vi "GetCircleResultValue.vi"(8 "error in (no error)":errorcluster, 9 "data":T2 {"ROI Descriptor out"."Contours"."Type" items=["No Selection", "Point", "Line", "Rectangle", "Oval", "Polygon", "Freehand Region", "Annulus", "Unused2", "Unused3", "Broken Line", "Freehand Line", "Rotated Rectangle"]; "ROI Descriptor out"."Contours"."Type" items=["No Selection", "Point", "Line", "Rectangle", "Oval", "Polygon", "Freehand Region", "Annulus", "Unused2", "Unused3", "Broken Line", "Freehand Line", "Rotated Rectangle"]}, 11 "Analysis_Circle_Parameter":T3={"ROI Descriptor"={"Global Rectangle"=[], "Contours"=[]}, "Options"={"Search  Direction"=0, "Edge Options"={"Edge Polarity"=0, "Kernel Size"=3, "Width"=3, "Minimum Edge Strength"=10.0, "Interpolation Type"=enum."Bilinear Fixed", "Data Processing Method"=enum."Average"}, "Show Search Area"=FALSE, "Show Search Lines"=FALSE, "Show Edges Found"=FALSE, "Show Result"=TRUE, "Search Area Color"=65280, "Search Lines Color"=255, "Edge Locations Color"=16776960, "Result Color"=16711680, "Overlay Group Name"=""}, "Circle Fit Options"={"Process"=enum."Get First Edge", "Step Size"=3.0, "Max Pixel Radius"=3}} {"Options"."Search  Direction" items=["Outside to Inside", "Inside to Outside"]; "Options"."Edge Options"."Edge Polarity" items=["All Edges", "Rising Edges", "Falling Edges"]; "Options"."Edge Options"."Minimum Edge Strength" format="%.2f"; "Options"."Edge Options"."Width" step=2; "Options"."Edge Options"."Kernel Size" step=2}) -> (0 "error out":errorcluster, 3 "ResultValues":string[](array[string]))   [LabVIEW 2019]
uses:
  Controls/Circle/Analysis_Circle_Parameter.ctl
  <vilib>/vision/Measure.llb/Edge Options.ctl
  <vilib>/vision/Measure.llb/Edge Polarity.ctl
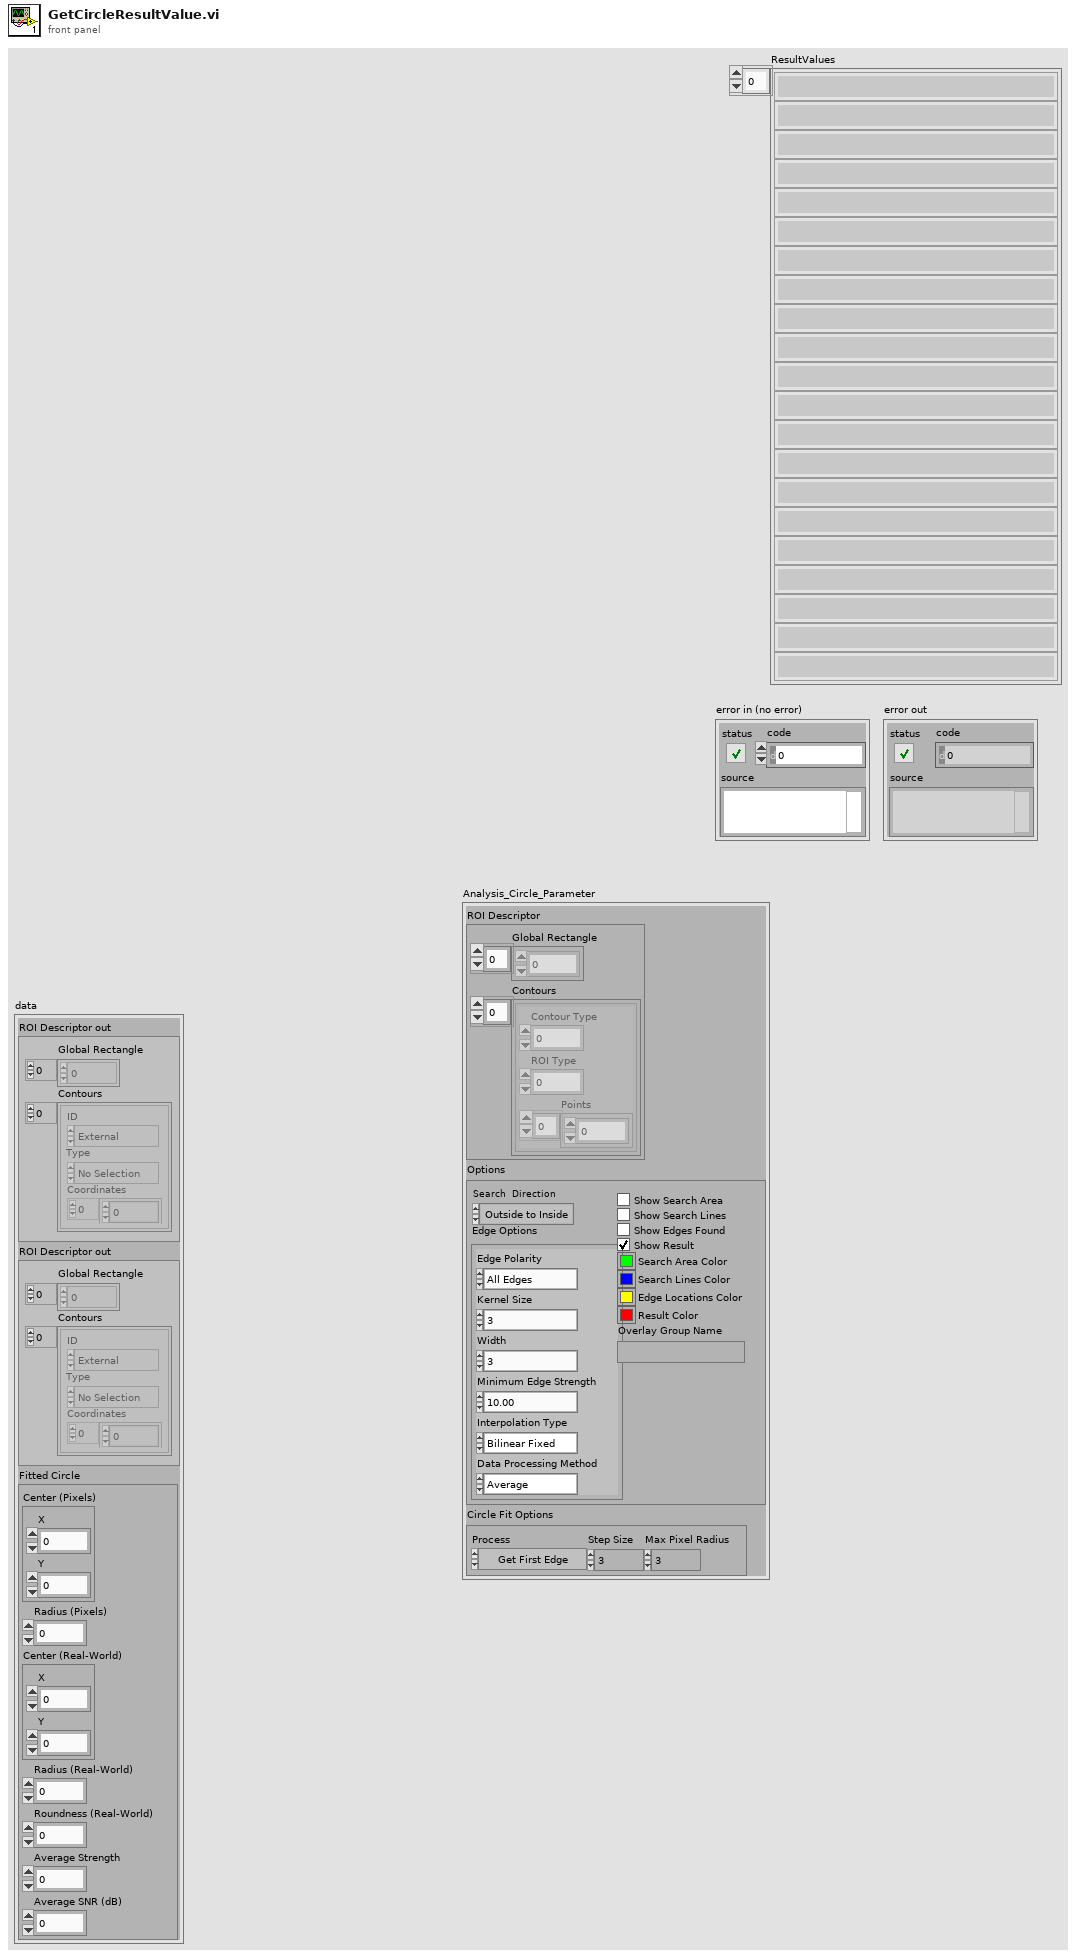
[diagram p1: front panel]
types:
  T1 = typedef "ROI Descriptor" = cluster{"Global Rectangle":i32[], "Contours":cluster{"ID":enum32{"External", "Internal"}, "Type":u32, "Coordinates":i32[]}[]}
  T2 = cluster{"ROI Descriptor out":T1, "ROI Descriptor out":T1, "Fitted Circle":cluster{"Center (Pixels)":cluster{"X":sgl, "Y":sgl}, "Radius (Pixels)":dbl, "Center (Real-World)":cluster{"X":sgl, "Y":sgl}, "Radius (Real-World)":dbl, "Roundness (Real-World)":dbl, "Average Strength":dbl, "Average SNR (dB)":dbl}}
  T3 = typedef "Analysis_Circle_Parameter.ctl" = cluster{"ROI Descriptor":cluster{"Global Rectangle":i32[], "Contours":cluster{"Contour Type":u32, "ROI Type":u32, "Points":i32[]}[]}, "Options":cluster{"Search  Direction":u32, "Edge Options":T4, "Show Search Area":bool, "Show Search Lines":bool, "Show Edges Found":bool, "Show Result":bool, "Search Area Color":u32, "Search Lines Color":u32, "Edge Locations Color":u32, "Result Color":u32, "Overlay Group Name":string}, "Circle Fit Options":cluster{"Process":enum16{"Get First Edge", "Get First + Last Edge", "Get All Edges", "Get Best Edge"}, "Step Size":dbl, "Max Pixel Radius":i32}}
  T4 = typedef "Edge Options.ctl" = cluster{"Edge Polarity":T5, "Kernel Size":u32, "Width":u32, "Minimum Edge Strength":sgl, "Interpolation Type":enum32{"Zero Order", "Bilinear", "Quadratic", "Cubic", "Bilinear Fixed"}, "Data Processing Method":enum32{"Average", "Median"}}
  T5 = typedef "Edge Polarity.ctl" = u32
  T6 = cluster{"Center (Pixels)":cluster{"X":sgl, "Y":sgl}, "Radius (Pixels)":dbl, "Center (Real-World)":cluster{"X":sgl, "Y":sgl}, "Radius (Real-World)":dbl, "Roundness (Real-World)":dbl, "Average Strength":dbl, "Average SNR (dB)":dbl}
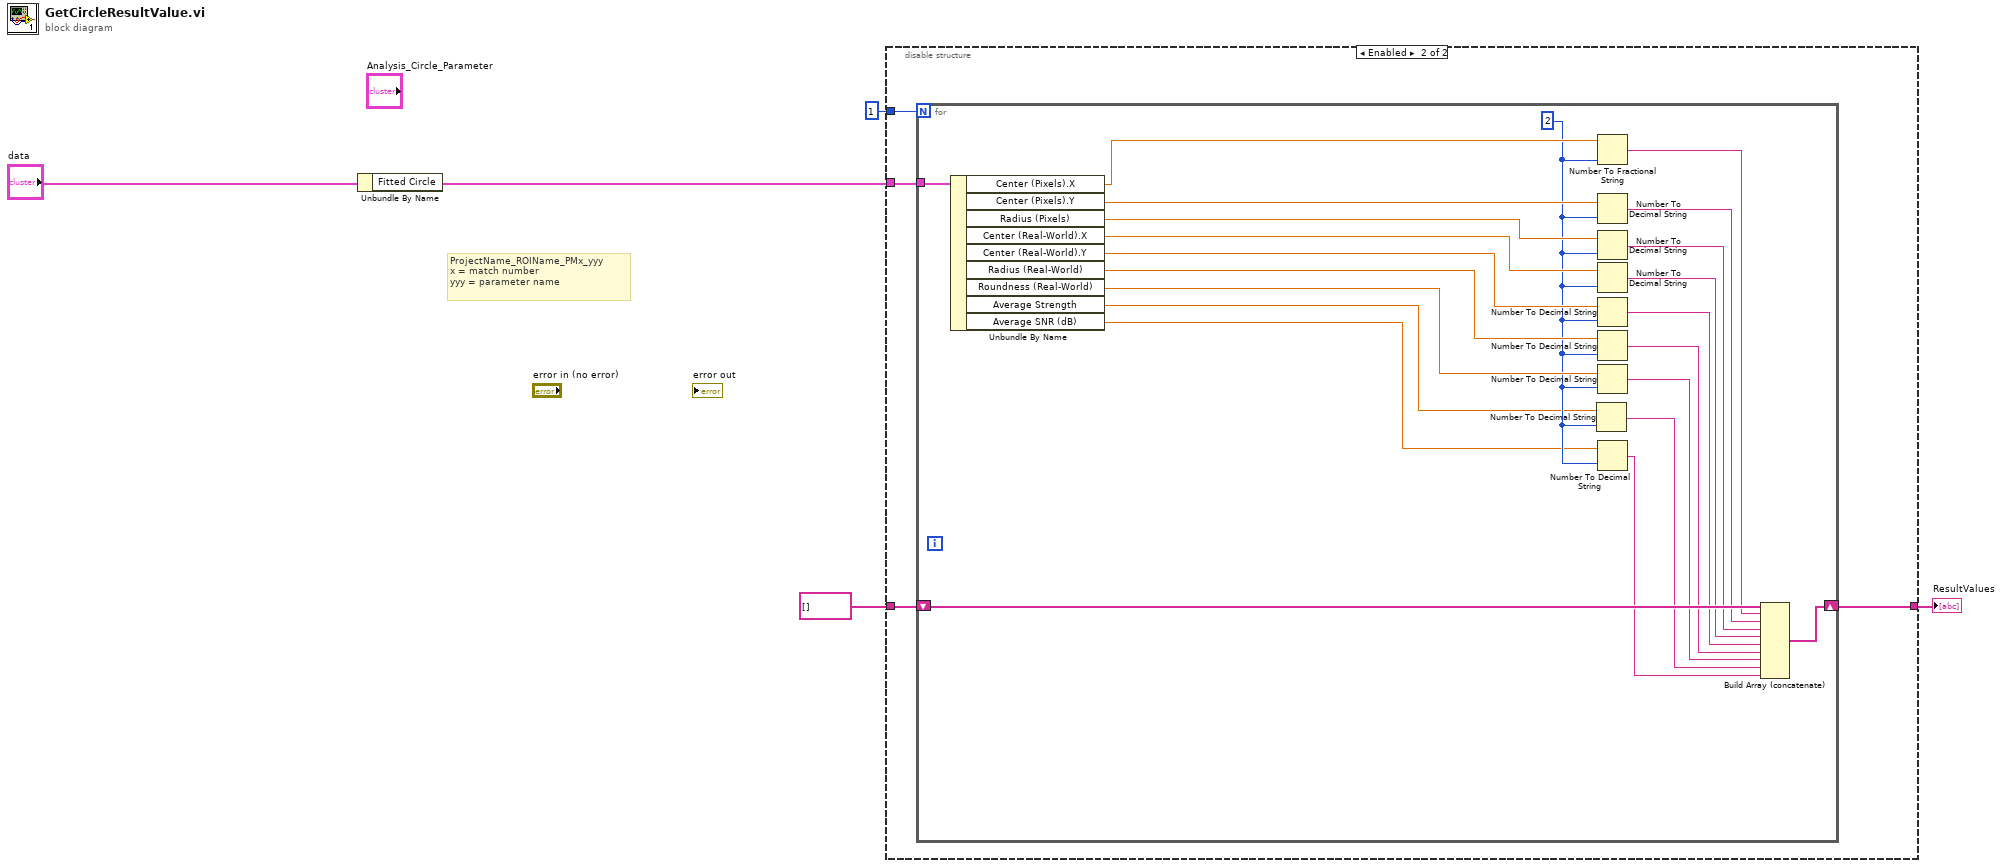
[diagram p0: block diagram]
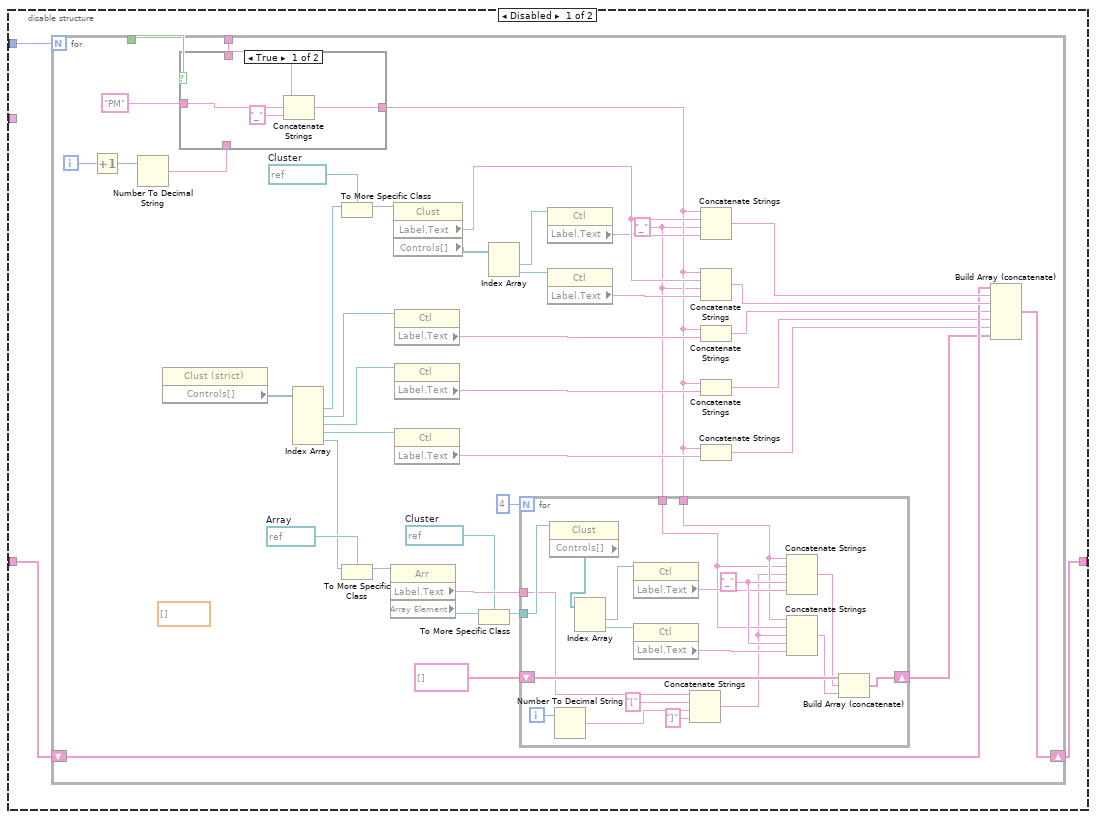
[diagram p2: hidden frame]
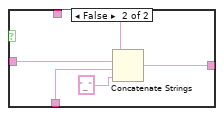
[diagram p3: hidden frame]
diagram:
  # "ProjectName_ROIName_PMx_yyy\nx = match number\nyyy = parameter name"
  n1 = Unbundle By Name("data") -> ("Fitted Circle"=w2:T6)
  n2 = disable-structure shown="Enabled" {
    disable-tunnel: 1 ("Number of Matches Requested") -> [w9 w83]
    disable-tunnel: string[] [] -> [w8 w82]
    disable-tunnel: [w7 w81] -> w4
    disable-tunnel: w2 -> [_ w80]
    frame Disabled {
      n3 = for {
        N: w9 -> [_]
        tunnel: _ -> [w31]
        shift-right: [w33] -> w7
        shift-left: w8 -> [w34]
        tunnel: [w32] -> w6
        i -> [w37]
        w16 = refnum<vi> refnum  # Cluster
        (unwired) dbl[] []
        w21 = refnum<vi> refnum  # Array
        w12 = "_" ("string")
        w47 = refnum<vi> refnum  # Cluster
        n4 = Increment(x=w37) -> (x+1=w36:i32)
        n5 = Number To Decimal String(number=w36) -> (decimal integer string=w30:string)  [unwired: 1 in]
        n6 = property class="Clust (strict)"() -> (reference=w51:refnum<vi>, "Controls[]"=w50:refnum<vi>[])  [unwired: 1 in, 2 out]
        n7 = case shown="True" w32 {
          tunnel: w31 -> [w74 w79]
          tunnel: w30 -> [_ w76]
          tunnel: [w73 w78] -> w13
          tunnel: "PM" ("string") -> [w72 w75]
          frame True {
            n8 = Concatenate Strings(w74, w72, "_" ("string")) -> (w73:string)
          }
          frame False {
            n9 = Concatenate Strings(w79, w75, w76, "_" ("string")) -> (w78:string)
          }
        }
        n10 = Index Array(array=w50) -> (element #1=w49:refnum<vi>, element #2=w28:refnum<vi>, element #3=w27:refnum<vi>, element #4=w40:refnum<vi>, element #5=w20:refnum<vi>)  [unwired: 5 in]
        n11 = To More Specific Class(target class=w47, reference=w49) -> (specific class reference=w48:refnum<vi>)  [unwired: 1 in, 1 out]
        n12 = To More Specific Class(target class=w21, reference=w20) -> (specific class reference=w19:refnum<vi>)  [unwired: 1 in, 1 out]
        n13 = property class="Arr"(reference=w19) -> ("Label.Text"=w18:string, "Array Element"=w15:refnum<vi>)  [unwired: 1 in, 2 out]
        n14 = property class="Clust"(reference=w48) -> ("Label.Text"=w43:string, "Controls[]"=w46:refnum<vi>[])  [unwired: 1 in, 2 out]
        n15 = property class="Ctl"(reference=w28) -> ("Label.Text"=w26:string)  [unwired: 1 in, 2 out]
        n16 = property class="Ctl"(reference=w27) -> ("Label.Text"=w25:string)  [unwired: 1 in, 2 out]
        n17 = property class="Ctl"(reference=w40) -> ("Label.Text"=w35:string)  [unwired: 1 in, 2 out]
        n18 = To More Specific Class(target class=w16, reference=w15) -> (specific class reference=w14:refnum<vi>)  [unwired: 1 in, 1 out]
        n19 = Index Array(array=w46) -> (element #1=w45:refnum<vi>, element #2=w44:refnum<vi>)  [unwired: 2 in]
        n20 = for {
          N: 4 -> [_]
          tunnel: w18 -> [w56]
          tunnel: w14 -> [w70]
          tunnel: w13 -> [w63]
          tunnel: w12 -> [w62]
          shift-right: [w58] -> w10
          shift-left: string[] [] -> [w61]
          i -> [w57]
          w69 = "_" ("string")
          n21 = property class="Clust"(reference=w70) -> ("Controls[]"=w64:refnum<vi>[])  [unwired: 1 in, 2 out]
          n22 = Number To Decimal String(number=w57) -> (decimal integer string=w54:string)  [unwired: 1 in]
          n23 = Index Array(array=w64) -> (element #1=w65:refnum<vi>, element #2=w66:refnum<vi>)  [unwired: 2 in]
          n24 = property class="Ctl"(reference=w65) -> ("Label.Text"=w67:string)  [unwired: 1 in, 2 out]
          n25 = property class="Ctl"(reference=w66) -> ("Label.Text"=w68:string)  [unwired: 1 in, 2 out]
          n26 = Concatenate Strings(w56, "[" ("string"), w54, "]" ("string")) -> (w52:string)
          n27 = Concatenate Strings(w63, w62, w52, w69, w67) -> (w60:string)
          n28 = Concatenate Strings(w63, w62, w52, w69, w68) -> (w59:string)
          n29 = Build Array (concatenate)(w61, w60, w59) -> (w58:string[])
        }
        n30 = property class="Ctl"(reference=w45) -> ("Label.Text"=w42:string)  [unwired: 1 in, 2 out]
        n31 = property class="Ctl"(reference=w44) -> ("Label.Text"=w41:string)  [unwired: 1 in, 2 out]
        n32 = Concatenate Strings(w13, w43, w12, w42) -> (w39:string)
        n33 = Concatenate Strings(w13, w43, w12, w41) -> (w38:string)
        n34 = Concatenate Strings(w13, w26) -> (w22:string)
        n35 = Concatenate Strings(w13, w25) -> (w23:string)
        n36 = Concatenate Strings(w13, w35) -> (w24:string)
        n37 = Build Array (concatenate)(w34, w39, w38, w22, w23, w24, w10) -> (w33:string[])
      }
    }
    frame Enabled {
      n38 = for {
        N: w83 -> [_]
        shift-right: [w103] -> w81
        shift-left: w82 -> [w104]
        tunnel: w80 -> [w105]
        w88 = 2
        n39 = Unbundle By Name(w105) -> ("Center (Pixels).X"=w102:sgl, "Center (Pixels).Y"=w94:sgl, "Radius (Pixels)"=w93:dbl, "Center (Real-World).X"=w92:sgl, "Center (Real-World).Y"=w91:sgl, "Radius (Real-World)"=w90:dbl, "Roundness (Real-World)"=w89:dbl, "Average Strength"=w87:dbl, "Average SNR (dB)"=w86:dbl)
        n40 = Number To Decimal String(number=w87, width (-)=w88) -> (decimal integer string=w85:string)
        n41 = Number To Fractional String(number=w102, precision (6)=w88) -> (F-format string=w101:string)  [unwired: 2 in]
        n42 = Number To Decimal String(number=w94, width (-)=w88) -> (decimal integer string=w100:string)
        n43 = Number To Decimal String(number=w93, width (-)=w88) -> (decimal integer string=w99:string)
        n44 = Number To Decimal String(number=w92, width (-)=w88) -> (decimal integer string=w98:string)
        n45 = Number To Decimal String(number=w91, width (-)=w88) -> (decimal integer string=w97:string)
        n46 = Number To Decimal String(number=w90, width (-)=w88) -> (decimal integer string=w96:string)
        n47 = Number To Decimal String(number=w89, width (-)=w88) -> (decimal integer string=w95:string)
        n48 = Number To Decimal String(number=w86, width (-)=w88) -> (decimal integer string=w84:string)
        n49 = Build Array (concatenate)(w104, w101, w100, w99, w98, w97, w96, w95, w85, w84) -> (w103:string[])
      }
    }
  }
  "ResultValues" <- w4
